vi "Untitled 2.vi"() -> ()   [LabVIEW 2019]
uses:
  <vilib>/userDefined/High Color/IMAQdx.ctl
  <vilib>/vision/driver/NI_Vision_Acquisition_Software.lvlib
  <vilib>/vision/NI_Vision_Development_Module.lvlib
panel:
  out "Standard  Deviation":sgl format="%.2f"
  out "Buffer Number Out":u32
  in  "Stop Button":bool
  out "error out":errorcluster
  out "Image":T1(plugin-control)
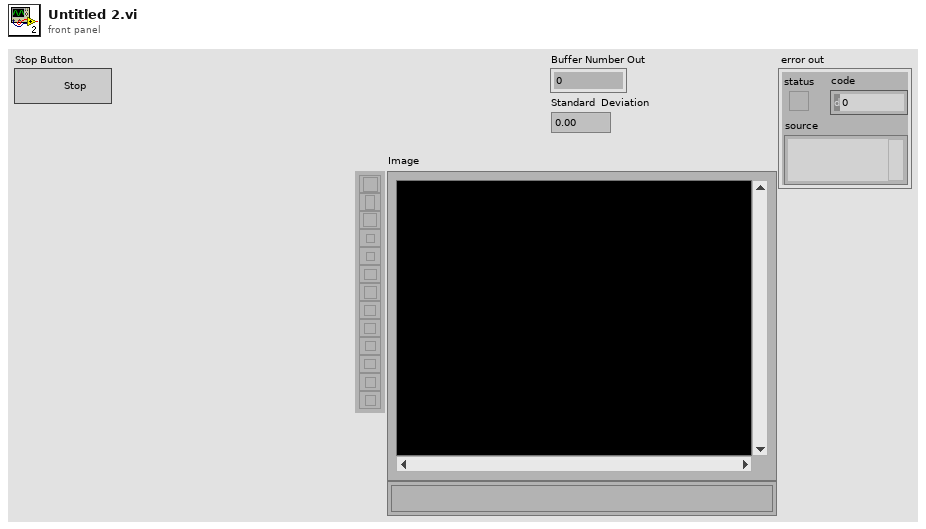
[diagram p1: front panel]
types:
  T1 = typedef "IMAQ Image.ctl" = refnum<image>
  T2 = typedef "Image Type" = u32
  T3 = typedef "IMAQdx.ctl" = refnum<k21>
  T4 = enum32{"Differentiation", "Gradient", "Prewitt", "Roberts", "Sigma", "Sobel"}
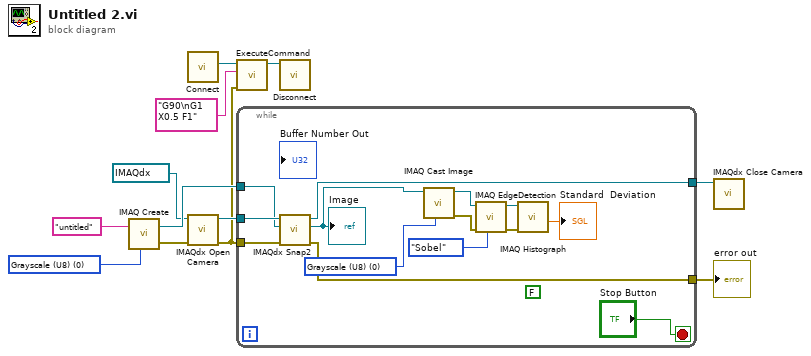
[diagram p0: block diagram]
diagram:
  w5 = T2 0 items=["Grayscale (U8)", "Grayscale (I16)", "Grayscale (SGL)", "Complex (CSG)", "RGB (U32)", "HSL (U32)", "RGB (U64)", "Grayscale (U16)"] ("Image Type")
  n1 = call "IMAQ Create"("Image Name"="untitled", "Image Type"=w5) -> ("New Image"=w12:T1, "error out"=w7:errorcluster)  [unwired: 3 in]
  n2 = call "Connect.vi"() -> ("controller"=w4:refnum<k24>)  [unwired: 10 in, 1 out]
  n3 = call <vilib>:"IMAQdx Open Camera.vi"("error in"=w7, "Session In"=T3 "cam1") -> ("error out"=w2:errorcluster, "Session Out"=w6:T3)  [unwired: 8 in]
  n4 = call "ExecuteCommand.vi"("error in (no error)"=w2, "Command Code"="G90\nG1 X0.5 F1", "controller in"=w4) -> ("controller out"=w1:refnum<k24>)  [unwired: 6 in, 2 out]
  n5 = while {
    tunnel: w6 -> [w26]
    tunnel: w12 -> [w25]
    tunnel: [w23] -> w10
    tunnel: [w22] -> w8
    tunnel: w2 -> [w21]
    stop <- "Stop Button" stop-if-true
    w13 = T2 0 items=["Grayscale (U8)", "Grayscale (I16)", "Grayscale (SGL)", "Complex (CSG)", "RGB (U32)", "HSL (U32)", "RGB (U64)", "Grayscale (U16)"] ("Image Type")
    (unwired) FALSE ("Wait for Next Buffer? (Yes)")
    n6 = call <vilib>:"IMAQdx Snap2.vi"("error in"=w21, "Image In"=w25, "Session In"=w26) -> ("error out"=w23:errorcluster, "Image Out"=w17:T1, "Session Out"=w22:T3)  [unwired: 6 in]
    "Image" <- w17
    n7 = call "IMAQ Cast Image"("Image Type"=w13, "Image Src"=w17) -> ("error out"=w18:errorcluster, "Image Dst Out"=w16:T1)  [unwired: 8 in]
    n8 = call "IMAQ EdgeDetection"("Method"=T4."Sobel", "error in (no error)"=w18, "Image Src"=w16) -> ("error out"=w20:errorcluster, "Image Dst Out"=w15:T1)  [unwired: 7 in]
    n9 = call "IMAQ Histograph"("error in (no error)"=w20, "Image"=w15) -> ("Standard  Deviation"=→"Standard  Deviation":sgl)  [unwired: 6 in, 3 out]
  }
  "error out" <- w10
  n10 = call "Disconnect.vi"("controller"=w1) -> ()  [unwired: 10 in, 1 out]
  n11 = call <vilib>:"IMAQdx Close Camera.vi"("Session In"=w8) -> ()  [unwired: 10 in, 1 out]
